vi "API Color Sensor Dev Init.vi"(10 "PortName":i32) -> (3 "DevInit Return value":bool)   [LabVIEW 2011, in "API ColorSensor.lvlib"]
uses:
  API ColorSensor.lvlib
  ColorSensor.dll
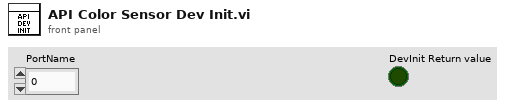
[diagram p1: front panel]
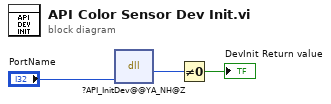
[diagram p0: block diagram]
diagram:
  n1 = dll-call lib="PTH1pabs CUsers\nAdministratorDesktop可重构机电平台项目DemoLabView基础APIColorSensor.dll" fn="?API_InitDev@@YA_NH@Z"("PortName"="PortName") -> ("返回类型"=w2:i32)  [unwired: 4 in, 2 out]
  n2 = Not Equal To 0?(x=w2) -> (x != 0?=→"DevInit Return value":bool)
